vi "Write Tasks names.vi"(8 "error in (no error)":errorcluster caption="entrée d'erreur (pas d'erreur)", 10 "Tasks names":string[](array[string]), 11 "DAQmxTaskContainer en entrée":refnum<class "DAQmxTaskContainer.lvclass">) -> (0 "error out":errorcluster caption="sortie d'erreur", 3 "DAQmxTaskContainer en sortie":refnum<class "DAQmxTaskContainer.lvclass">)   [LabVIEW 2015, in "DAQmxTaskContainer.lvclass"]
uses:
  DAQmxTaskContainer.lvclass
  DAQmxTaskContainer.lvclass/DAQmxTaskContainer.ctl
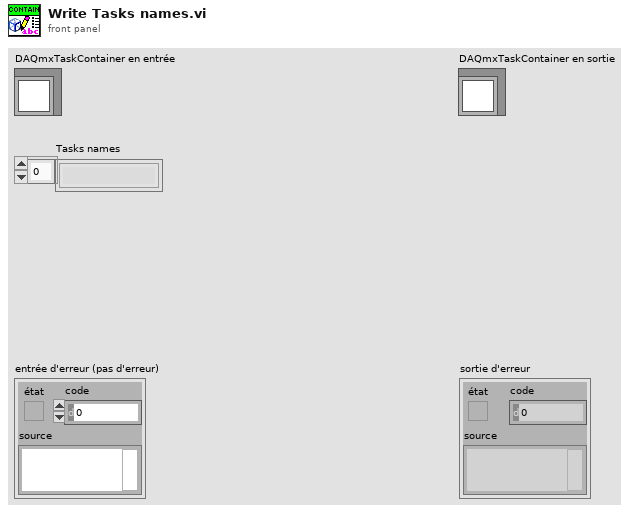
[diagram p1: front panel]
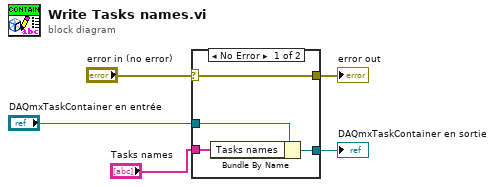
[diagram p0: block diagram]
diagram:
  n1 = case shown="No Error" "error in (no error)" {
    selector: "error in (no error)" -> [w9 w10]
    tunnel: [w9 w10] -> w4
    tunnel: [w7 w11] -> w2
    tunnel: "DAQmxTaskContainer en entrée" -> [w8 w11]
    tunnel: "Tasks names" -> [w6 _]
    frame No Error {
      n2 = Bundle By Name(cluster=w8, "Tasks names"=w6) -> (w7:refnum<class "DAQmxTaskContainer.lvclass">)
    }
    frame Error {
    }
  }
  "error out" <- w4
  "DAQmxTaskContainer en sortie" <- w2
